vi "Load Config.vi"(8 "error in (no error)":errorcluster, 11 "Config-INI in":refnum<class "Config-INI.lvclass">) -> (0 "error out":errorcluster, 2 "Elements":T1[](array[typedef]), 3 "Config-INI out":refnum<class "Config-INI.lvclass">)   [LabVIEW 2020, in "CDM-Config.lvlib" / "Config-INI.lvclass"]
uses:
  Config-INI.lvclass
  <vilib>/Utility/config.llb/NI_LVConfig.lvlib
  df3b4445-68e4-4fb6-9c5e-98fcdeb0131b.vi
  <vilib>/Utility/config.llb/Read Key (String).vi
  Meta Data.ctl
  CDM-Config.lvlib
  Config Element.ctl
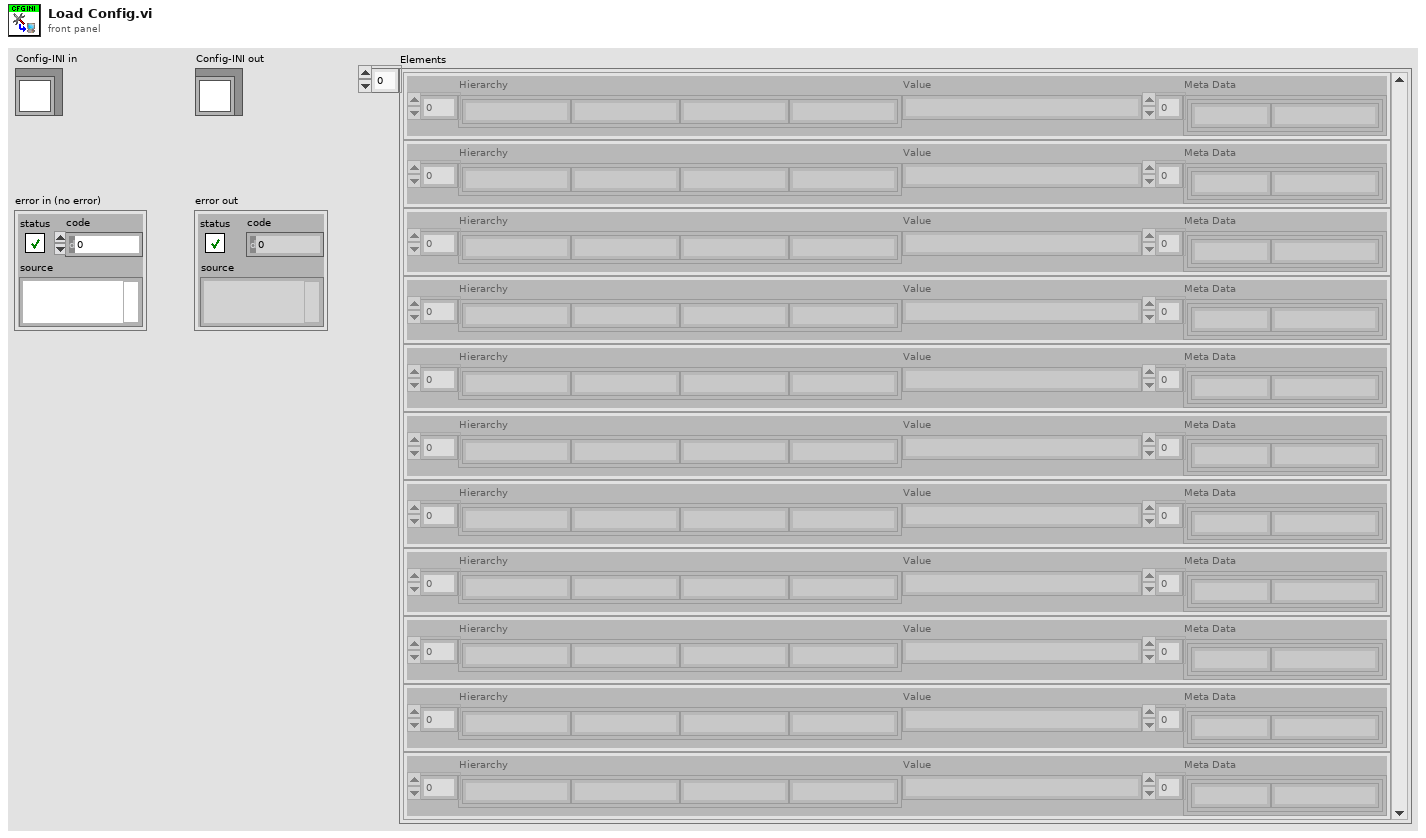
[diagram p1: front panel]
types:
  T1 = typedef "CDM-Config.lvlib/Config Element.ctl" = cluster{"Hierarchy":string[], "Value":string, "Meta Data":T2[]}
  T2 = typedef "CDM-Config.lvlib/Meta Data.ctl" = cluster{"Name":string, "Value":string}
  T3 = typedef "NI_LVConfig.lvlib/Config Data RefNum.ctl" = refnum<k1>
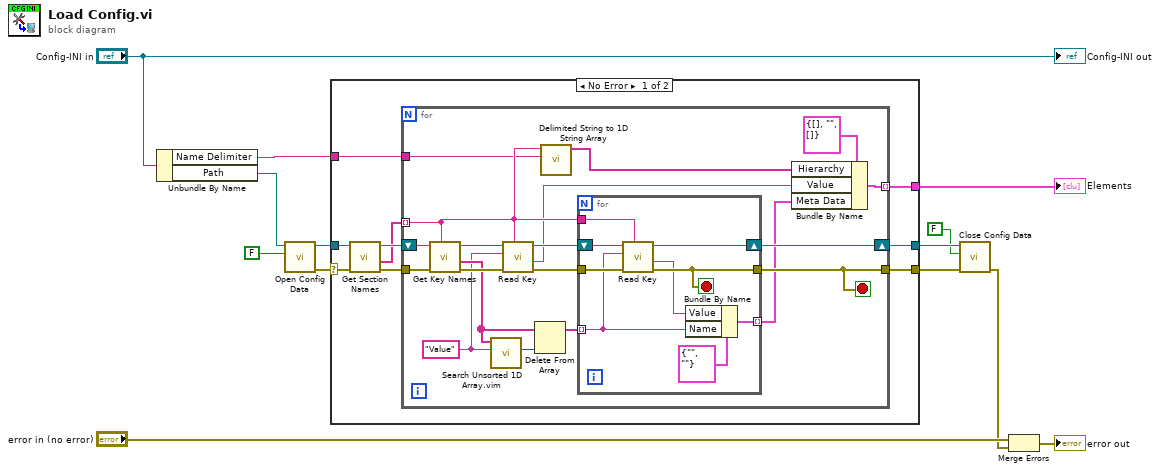
[diagram p0: block diagram]
diagram:
  n1 = Unbundle By Name("Config-INI in") -> ("Name Delimiter"=w3:string, "Path"=w12:path)
  n2 = call <vilib>:"Open Config Data.vi"("create file if necessary (T)"=FALSE, "configuration file path"=w12) -> ("error out"=w9:errorcluster, "refnum"=w10:T3)  [unwired: 7 in, 1 out]
  n3 = case shown="No Error" w9 {
    selector: w9 -> [w21 w51]
    tunnel: w10 -> [w22 w52]
    tunnel: [w17 w52] -> w8
    tunnel: [w16 w51] -> w6
    tunnel: w3 -> [w15 _]
    tunnel: [w14 _] -> w1
    frame No Error {
      n4 = call <vilib>:"Get Section Names.vi"("error in (no error)"=w21, "refnum"=w22) -> ("error out"=w20:errorcluster, "section names"=w18:string[], "refnum out"=w19:T3)  [unwired: 7 in]
      n5 = for {
        tunnel: w20 -> [w39]
        tunnel: w18 -> [w30] mode=indexing
        shift-right: [w36] -> w17
        shift-left: w19 -> [w40]
        tunnel: [w28] -> w16
        tunnel: w15 -> [w29]
        tunnel: [w23] -> w14 mode=indexing
        stop <- w28 stop-if-true
        w31 = "Value"
        n6 = call <vilib>:"Get Key Names.vi"("section"=w30, "error in (no error)"=w39, "refnum"=w40) -> ("error out"=w41:errorcluster, "key names"=w38:string[], "refnum out"=w34:T3)  [unwired: 5 in, 1 out]
        n7 = call "Search Unsorted 1D Array.vim"("element"=w31, "unsorted 1D array"=w38) -> ("index of element"=w37:i32)  [unwired: 9 in]
        n8 = call-poly <vilib>:"Read Key.vi"("section"=w30, "error in (no error)"=w41, "key"=w31, "refnum"=w34) -> ("error out"=w32:errorcluster, "value"=w25:string, "refnum out"=w33:T3)  [unwired: 4 in, 1 out]
        n9 = Delete From Array(array=w38, index=w37) -> (array with subset deleted=w35:string[])  [unwired: 1 in, 1 out]
        n10 = call <vilib>:"Delimited String to 1D String Array.vi"("delimiter"=w29, "delimited string"=w30) -> ("string array"=w26:string[])  [unwired: 9 in]
        n11 = for {
          shift-right: [w42] -> w36
          shift-left: w33 -> [w50]
          tunnel: w35 -> [w44] mode=indexing
          tunnel: w32 -> [w49]
          tunnel: w30 -> [w48]
          tunnel: [w47] -> w28
          tunnel: [w43] -> w24 mode=indexing
          stop <- w47 stop-if-true
          n12 = call-poly <vilib>:"Read Key.vi"("section"=w48, "error in (no error)"=w49, "key"=w44, "refnum"=w50) -> ("error out"=w47:errorcluster, "value"=w45:string, "refnum out"=w42:T3)  [unwired: 4 in, 1 out]
          n13 = Bundle By Name(cluster=T2 {"Name"="", "Value"=""} ("Meta Data"), "Value"=w45, "Name"=w44) -> (w43:T2)
        }
        n14 = Bundle By Name(cluster=T1 {"Hierarchy"=[], "Value"="", "Meta Data"=[]} ("Config Element"), "Hierarchy"=w26, "Value"=w25, "Meta Data"=w24) -> (w23:T1)
      }
    }
    frame Error {
    }
  }
  "Elements" <- w1
  n15 = call <vilib>:"Close Config Data.vi"("error in (no error)"=w6, "write file if changed (T)"=FALSE, "refnum"=w8) -> ("error out"=w2:errorcluster)  [unwired: 7 in, 1 out]
  n16 = Merge Errors("error in (no error)", w2) -> (→"error out":errorcluster)
  "Config-INI out" <- "Config-INI in"
